vi "POP send DELE.vi"(3 "error in":errorcluster, 4 "MSG number":i32, 5 "connection ID in":refnum<k5>) -> (0 "error out":errorcluster, 1 "DELE response":string="\r\n", 2 "connection ID out":refnum<k5>)   [LabVIEW 2012]
doc: "This low-level POP VI sends the \"DELE\" command to a mail server, instructing it to delete the specified message from its user's account."
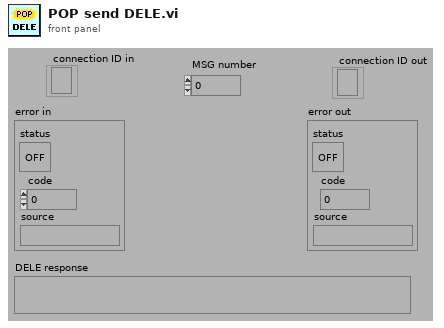
[diagram p1: front panel]
types:
  T1 = enum16{"Standard", "Buffered", "CRLF", "Immediate"}
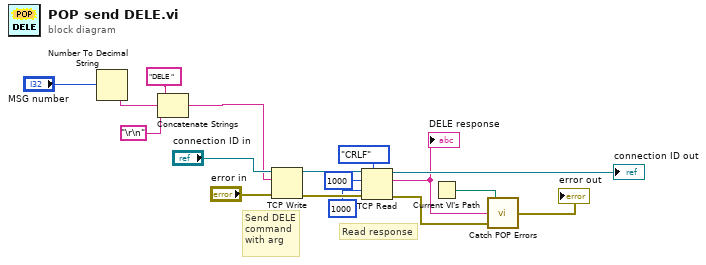
[diagram p0: block diagram]
diagram:
  # "Read response"
  # "Send DELE\ncommand\nwith arg"
  n1 = Number To Decimal String(number="MSG number") -> (decimal integer string=w5:string)  [unwired: 1 in]
  n2 = Concatenate Strings("DELE ", w5, "\r\n") -> (w8:string)
  n3 = TCP Write(connection ID="connection ID in", data in=w8, error in (no error)="error in") -> (connection ID out=w16:refnum<k5>, error out=w15:errorcluster)  [unwired: 1 in, 1 out]
  n4 = TCP Read(connection ID=w16, bytes to read=1000, error in (no error)=w15, 7:T1."CRLF" ("mode (standard)"), 9:1000 ("timeout ms (25000)")) -> (connection ID out=→"connection ID out":refnum<k5>, data out=w3:string, error out=w2:errorcluster)
  "DELE response" <- w3
  n5 = Current VI's Path() -> (path=w4:path)
  n6 = call "Catch POP Errors.vi"("error in"=w2, "POP server response"=w3, "Caller Path"=w4) -> ("error out"=→"error out":errorcluster)
